vi "CE Estimate measurement time.vi"(11 "CE measurement":T1={"Signal frequencies (Hz) T"=[1000.0], "Signal amplitudes (V) T"=[0.707], "Sampling frequencies (Hz) T"=[10000000.0], "Record lengths (multiples of periods) T"=[10000.0], "TWM data root directory"=path "", "TWM mreasurements directories"=[], "Calculate RMS from samples"=FALSE, "Algorithm to use"="TWM-WFFT", "Quantity to read"="TWM-WFFT", "Settle down after AC source change (s) T"=1.0, "Skip PJVS setup"=FALSE, "Measurement template file"=path "", "Row of START keyword T"=0, "Row of STOP keyword T"=0, "Measurement template line T"=[], "Switch position T"=[10000.0], "FR fit mat file T"=path "", "Recalculate-skip already calculated"=FALSE} {"Switch position T" format="%#_3p"; "Record lengths (multiples of periods) T" format="%#_3p"; "Sampling frequencies (Hz) T" format="%#_3p"; "Signal amplitudes (V) T" format="%#_3p"; "Signal frequencies (Hz) T" format="%#_3p"}) -> (1 "Estimate as formatted text":string, 3 "Estimate of measurement time (s)":dbl)   [LabVIEW 2020]
doc: "Estimates the total measurement time based on the measurement settings and devices settings."
uses:
  CE Measurement/Type definitions/CE measurement.ctl
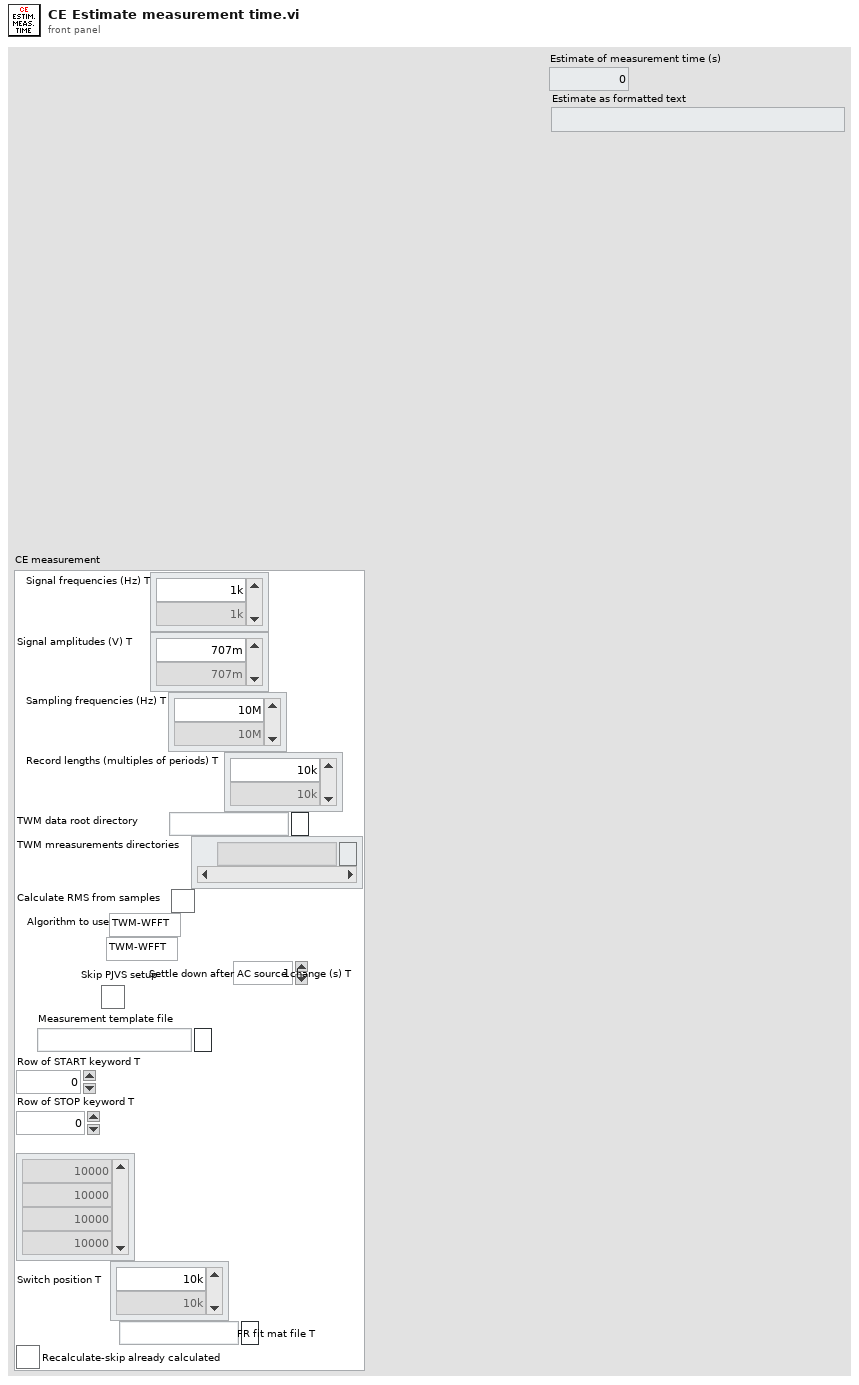
[diagram p1: front panel]
types:
  T1 = typedef "CE measurement.ctl" = cluster{"Signal frequencies (Hz) T":dbl[], "Signal amplitudes (V) T":dbl[], "Sampling frequencies (Hz) T":dbl[], "Record lengths (multiples of periods) T":dbl[], "TWM data root directory":path, "TWM mreasurements directories":path[], "Calculate RMS from samples":bool, "Algorithm to use":string, "Quantity to read":string, "Settle down after AC source change (s) T":dbl, "Skip PJVS setup":bool, "Measurement template file":path, "Row of START keyword T":i32, "Row of STOP keyword T":i32, "Measurement template line T":i32[], "Switch position T":dbl[], "FR fit mat file T":path, "Recalculate-skip already calculated":bool}
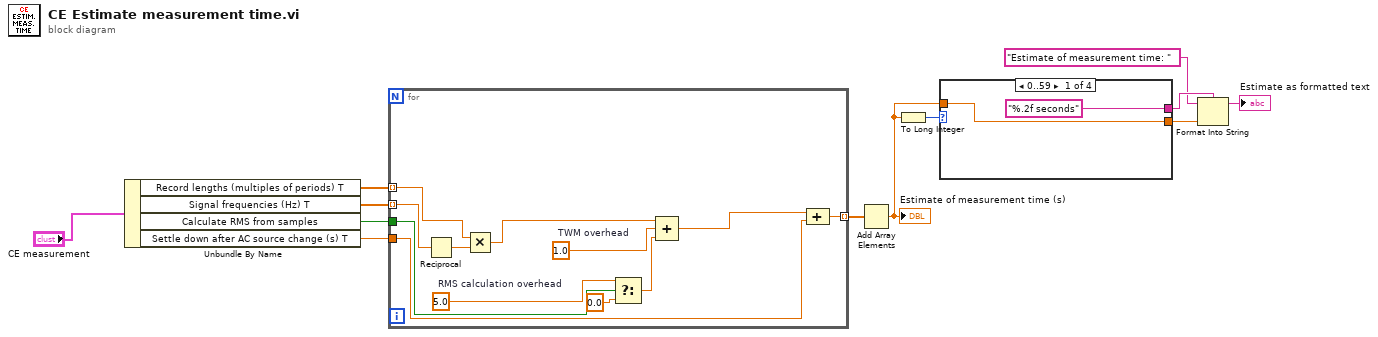
[diagram p0: block diagram]
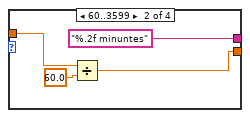
[diagram p2: hidden frame]
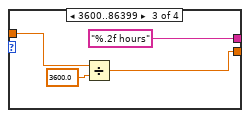
[diagram p3: hidden frame]
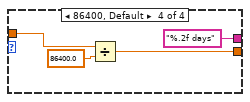
[diagram p4: hidden frame]
diagram:
  n1 = Unbundle By Name("CE measurement") -> ("Record lengths (multiples of periods) T"=w2:dbl[], "Signal frequencies (Hz) T"=w3:dbl[], "Calculate RMS from samples"=w4:bool, "Settle down after AC source change (s) T"=w5:dbl)
  n2 = for {
    tunnel: w3 -> [w24] mode=indexing
    tunnel: w2 -> [w22] mode=indexing
    tunnel: [w14] -> w12 mode=indexing
    tunnel: w4 -> [w19]
    tunnel: w5 -> [w15]
    w18 = 5.0  # RMS calculation overhead
    w21 = 1.0  # TWM overhead
    n3 = Reciprocal(x=w24) -> (1/x=w23:dbl)
    n4 = Multiply(x=w22, y=w23) -> (x*y=w20:dbl)
    n5 = Select(t=w18, s=w19, f=0.0 ("RMS calculation overhead")) -> (s? t:f=w16:dbl)
    n6 = Compound Arithmetic op=ADD(w20, w21, w16) -> (w13:dbl)
    n7 = Compound Arithmetic op=ADD(w13, w15) -> (w14:dbl)
  }
  n8 = Add Array Elements(numeric array=w12) -> (sum=w6:dbl)
  "Estimate of measurement time (s)" <- w6
  n9 = To Long Integer(number=w6) -> (32bit integer=w11:i32)
  n10 = case shown="0..59" w11 {
    tunnel: w6 -> [w25 w29 w33 w37]
    tunnel: [w25 w27 w32 w36] -> w10
    tunnel: ["%.2f seconds" ("format string") "%.2f minuntes" ("format string") "%.2f hours" ("format string") "%.2f days" ("format string")] -> w9
    frame 0..59 {
    }
    frame 60..3599 {
      n11 = Divide(x=w29, y=60.0) -> (x/y=w27:dbl)
    }
    frame 3600..86399 {
      n12 = Divide(x=w33, y=3600.0) -> (x/y=w32:dbl)
    }
    frame 86400, Default {
      n13 = Divide(x=w37, y=86400.0) -> (x/y=w36:dbl)
    }
  }
  n14 = Format Into String(format string=w9, initial string="Estimate of measurement time: ", w10) -> (resulting string=→"Estimate as formatted text":string)  [unwired: 1 in, 1 out]
